vi "FTW-Endpoint-Pipe-Construct.vi"(0 "FTW Endpoint":refnum<class "FTW-Endpoint.lvclass">, 7 "Requested Identity":string, 11 "error in":errorcluster) -> (4 "FTW Endpoint out":refnum<class "FTW-Endpoint.lvclass">, 8 "Actual Identity":string, 15 "error out":errorcluster)   [LabVIEW 2013, in "FTW-Endpoint.lvclass"]
uses:
  FTW-Endpoint.lvclass
  FTW-Endpoint.lvclass/FTW-Endpoint.ctl
panel:
  # "Inputs"
  # "Outputs"
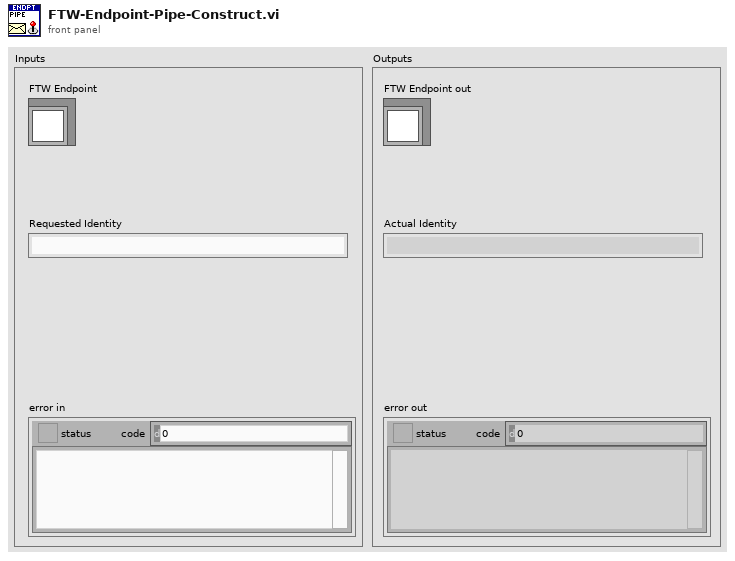
[diagram p1: front panel]
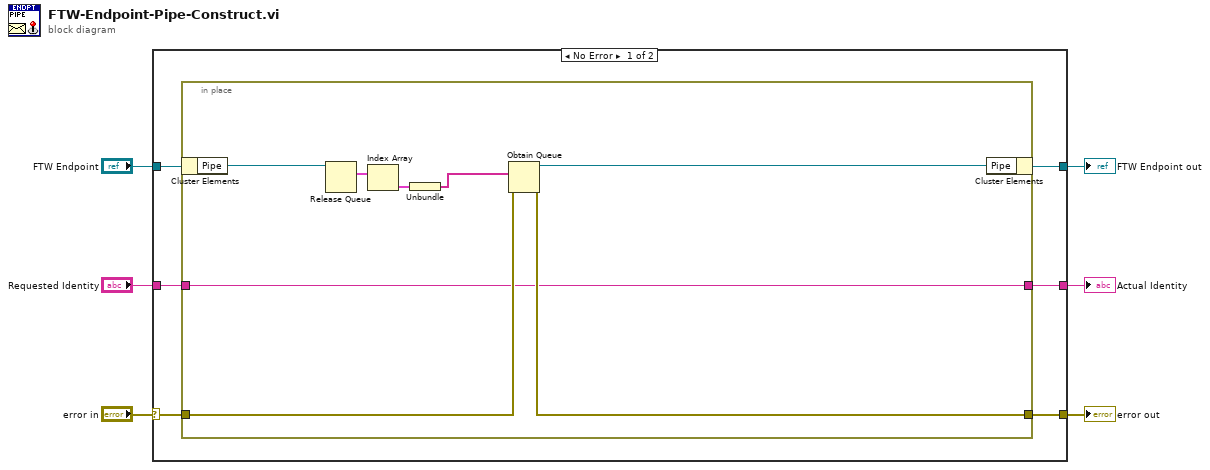
[diagram p0: block diagram]
diagram:
  n1 = case shown="No Error" "error in" {
    selector: "error in" -> [w10 w22]
    tunnel: [w8 w22] -> w6
    tunnel: [w9 w21] -> w4
    tunnel: "FTW Endpoint" -> [w12 w21]
    tunnel: "Requested Identity" -> [w11 _]
    tunnel: [w7 _] -> w1
    frame No Error {
      n2 = in-place {
        in-place-border: w11 -> [w13]
        in-place-border: w10 -> [w16]
        in-place-border: [w14] -> w8
        in-place-border: [w13] -> w7
        n3 = in-place-cluster #1(w12) -> ("Pipe"=w20:refnum<queue>)
        n4 = Release Queue(queue=w20) -> (remaining elements=w19:cluster{"Multipart Message":string[]}[])  [unwired: 2 in, 2 out]
        n5 = Index Array(array=w19) -> (element=w18:cluster{"Multipart Message":string[]})  [unwired: 1 in]
        n6 = Unbundle(w18) -> ("Multipart Message"=w17:string[])
        n7 = Obtain Queue(element data type=w17, error in (no error)=w16) -> (queue out=w15:refnum<queue>, error out=w14:errorcluster)  [unwired: 3 in, 1 out]
        n8 = in-place-cluster #1("Pipe"=w15) -> (w9:refnum<class "FTW-Endpoint.lvclass">)
      }
    }
    frame Error {
    }
  }
  "error out" <- w6
  "FTW Endpoint out" <- w4
  "Actual Identity" <- w1
